vi "VisualizeCHROMAAC.vi"() -> ()   [LabVIEW 2018, in "Visualization.lvlib" / "VisualizeAcPwr.lvclass"]
uses:
  VisualizeAcPwr.lvclass
  VisualizeBase/VisualizeBase_class/Requests/clUserEventType.ctl
  <vilib>/event_ctls.llb/usereventprio.ctl
  <vilib>/Utility/error.llb/Error Cluster From Error Code.vi
  <vilib>/ErrorRing/Error Ring.xnode
  VisualizeBase/VisualizeBase_class/VisualizeBase.lvclass
  <userlib>/NIST/NISTErrorLib/NISTErrorLib.lvlib
  AcPwr/AcPwrModule/AcPwrModule.lvlib
panel:
  in  "GraphAxis":u32[](array[numeric])=[0, 1, 1] max=1
  out "Chroma AC":waveform(dbl)[](graph)
  out "ErrorArray":errorcluster[](array[cluster])
  in  "QueueName":string="CHROMAACVQ"
  in  "btnStop":bool
  in  "btnReset":bool
  in  "btnClear":bool
  # "0=Left Axis and 1=Right Axis"
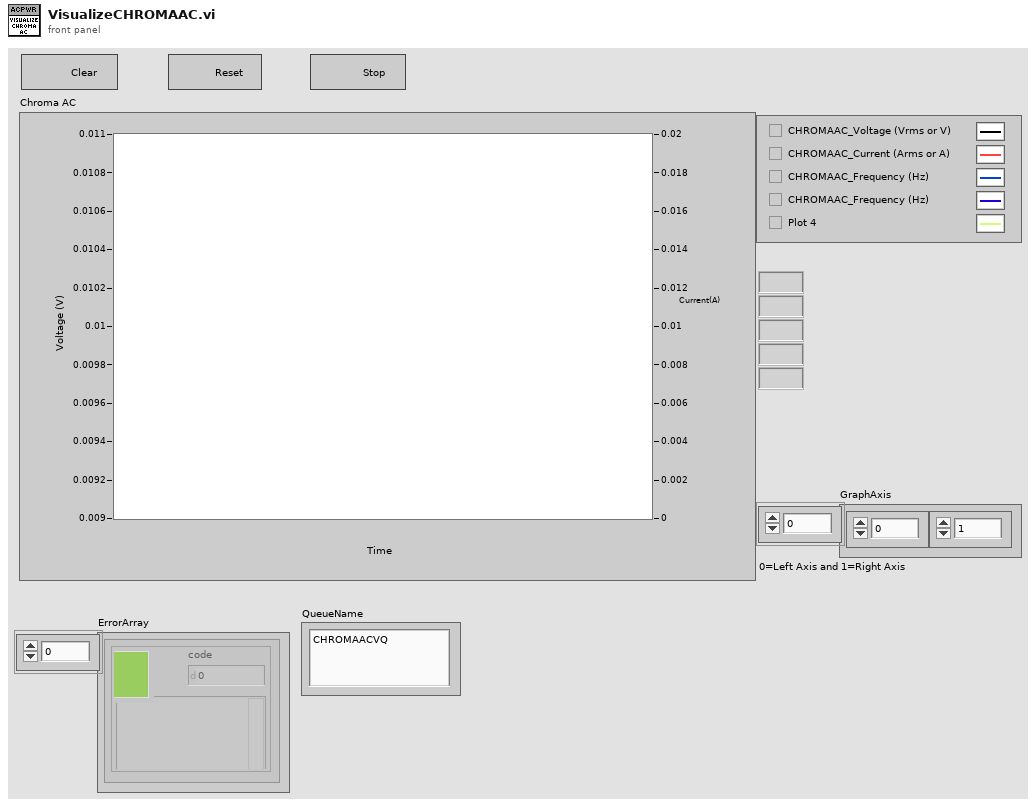
[diagram p1: front panel]
types:
  T1 = typedef "Visualization.lvlib/VisualizeBase.lvclass/clRequestEvents.ctl" = cluster{"StopRequest":refnum<user-event>, "ResetRequest":refnum<user-event>}
  T2 = typedef "AcPwrModule.lvlib/clBroadcastEvents.ctl" = cluster{"DidInit":refnum<user-event>, "StatusUpdate":refnum<user-event>, "ErrorReport":refnum<user-event>, "DidStop":refnum<user-event>, "PathToINI":refnum<user-event>, "Measurements":refnum<user-event>, "LoadConfigFile":refnum<user-event>}
  T3 = typedef "Visualization.lvlib/VisualizeBase.lvclass/clUserEventType.ctl" = cluster{"BusIndex":i8, "Data":variant}
  T4 = typedef "usereventprio.ctl" = enum32{"high priority", "normal priority"}
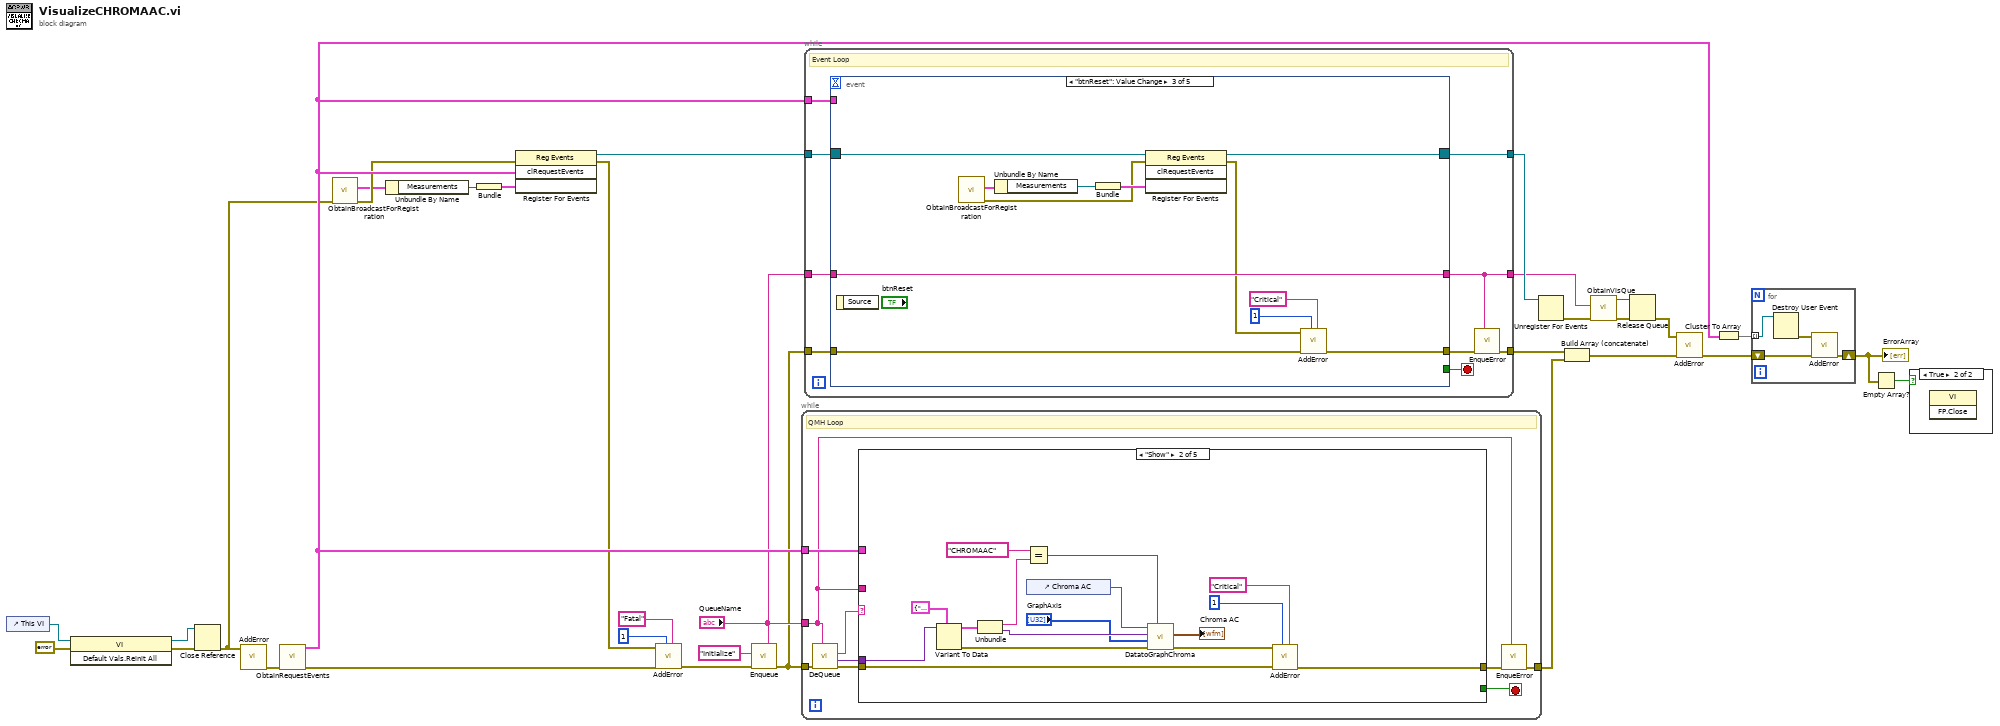
[diagram p0: block diagram]
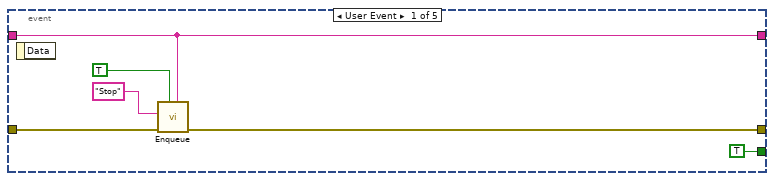
[diagram p2: hidden frame]
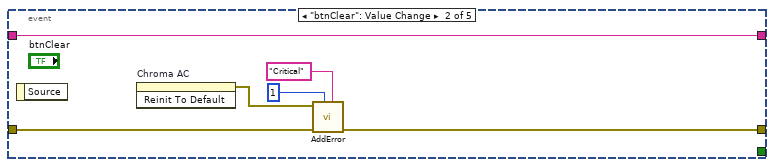
[diagram p3: hidden frame]
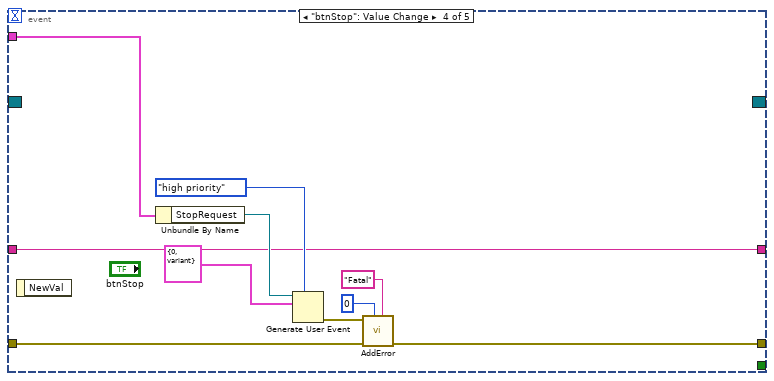
[diagram p4: hidden frame]
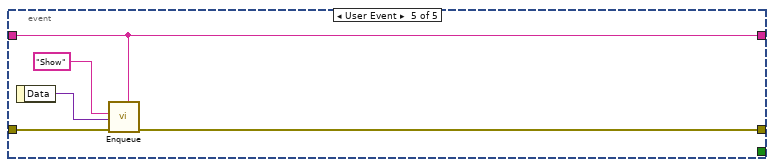
[diagram p5: hidden frame]
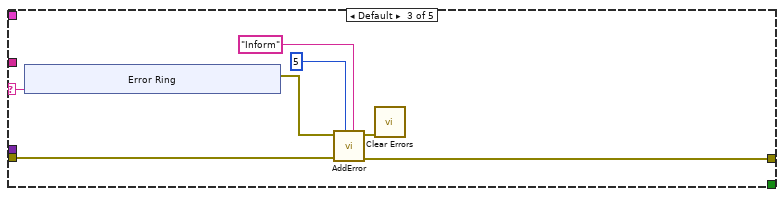
[diagram p8: hidden frame]
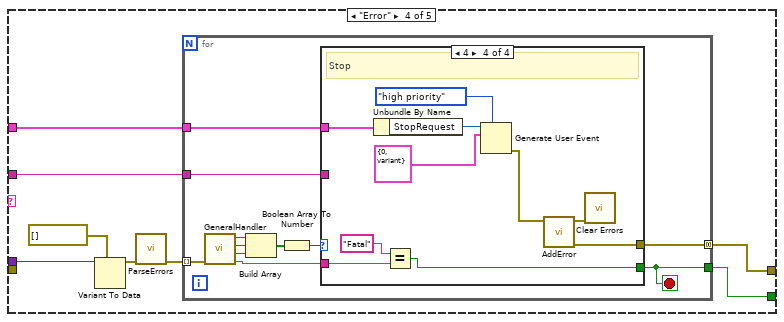
[diagram p9: hidden frame]
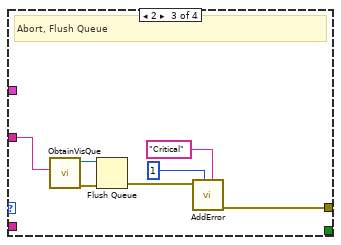
[diagram p12: hidden frame]
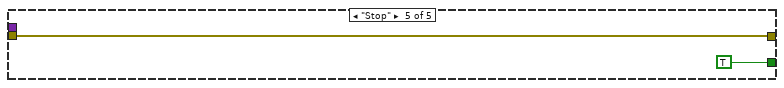
[diagram p13: hidden frame]
diagram:
  n1 = control-ref of="This VI"() -> (w16:refnum<vi>)
  n2 = invoke class="VI" method="Default Vals.Reinit All"(reference=w16, error in=errorcluster {"status"=FALSE, "code"=0, "source"=""} ("error in (no error)")) -> (reference out=w13:refnum<vi>, error out=w14:errorcluster)  [unwired: 1 in, 1 out]
  n3 = Close Reference(reference=w13, error in (no error)=w14) -> (error out=w11:errorcluster)
  n4 = call <userlib>:"AddError.vi"("error in (no error)"=w11) -> ("ErrorArray"=w31:errorcluster[])  [unwired: 9 in, 1 out]
  n5 = call "ObtainRequestEvents.vi"("Error"=w31) -> ("Error"=w4:errorcluster[], "clRequestEvents"=w20:T1)  [unwired: 9 in]
  n6 = call "ObtainBroadcastForRegistration.vi"("error in (no error)"=w11) -> ("error out"=w10:errorcluster, "clBroadcastEvents"=w9:T2)  [unwired: 9 in]
  n7 = Unbundle By Name(w9) -> ("Measurements"=w18:refnum<user-event>)
  n8 = Bundle("Measurements"=w18) -> (w17:cluster{"Measurements":refnum<user-event>})  [unwired: 1 in]
  n9 = register-events(error in=w10, w20, w17) -> (reference out=w32:refnum<event-registration>, error out=w1:errorcluster)  [unwired: 1 in]
  n10 = call <userlib>:"AddError.vi"("Severity"="Fatal" ("String"), "Priority"=u8 1, "ErrorArray"=w4, "error in (no error)"=w1) -> ("ErrorArray"=w3:errorcluster[])  [unwired: 6 in, 1 out]
  n11 = call "Enqueue.vi"("QueName"="QueueName", "Error"=w3, "Message"="Initialize") -> ("Error"=w2:errorcluster[])  [unwired: 8 in]
  n12 = while {
    tunnel: w2 -> [w42]
    tunnel: [w36] -> w27
    tunnel: "QueueName" -> [w34]
    tunnel: w20 -> [w35]
    stop <- w37 stop-if-true
    # "QMH Loop"
    n13 = call "DeQueue.vi"("QueName"=w34, "Error"=w42) -> ("Error"=w39:errorcluster[], "Data"=w40:variant, "Message"=w41:string)  [unwired: 7 in]
    n14 = case shown="\"Show\"" w41 {
      selector: w41 -> [_ _ w66 _ _]
      tunnel: w40 -> [_ w56 _ w81 _]
      tunnel: w39 -> [w43 w48 w64 _ w110]
      tunnel: [w43 w59 w63 w77 w110] -> w38
      tunnel: [_ _ _ w76 TRUE] -> w37
      tunnel: w35 -> [_ _ _ w75 _]
      tunnel: w34 -> [_ _ _ w74 _]
      frame "Initialize" {
      }
      frame "Show" {
        n15 = Variant To Data(type=cluster{string, "Data":variant} {"", "Data"=variant}, Variant=w56) -> (data=w57:cluster{string, "Data":variant}, error out=w51:errorcluster)  [unwired: 1 in]
        n16 = Unbundle(w57) -> (w55:string, "Data"=w52:variant)
        n17 = Equal?(x="CHROMAAC", y=w55) -> (x = y?=w49:bool)
        n18 = control-ref of="Chroma AC"() -> (w54:refnum<vi>)
        n19 = call "DatatoGraphChroma.vi"("Boolean"=w49, "error in (no error)"=w51, "Array 2"="GraphAxis", "Data"=w52, "WaveformChart in"=w54) -> ("error out"=w46:errorcluster, "Array"=→"Chroma AC":waveform(dbl)[])  [unwired: 3 in, 2 out]
        n20 = call <userlib>:"AddError.vi"("Severity"="Critical" ("String"), "Priority"=u8 1, "ErrorArray"=w48, "error in (no error)"=w46) -> ("ErrorArray"=w59:errorcluster[])  [unwired: 6 in, 1 out]
      }
      frame Default {
        n21 = xnode "Error Ring"("parameter 0"=w66) -> ("error out"=w65:errorcluster)
        n22 = call <userlib>:"AddError.vi"("Severity"="Inform" ("String"), "Priority"=u8 5, "ErrorArray"=w64, "error in (no error)"=w65) -> ("ErrorArray"=w63:errorcluster[], "error out"=w62:errorcluster)  [unwired: 6 in]
        n23 = call <vilib>:"Clear Errors.vi"("error in (no error)"=w62) -> ()  [unwired: 5 in, 2 out]
      }
      frame "Error" {
        n24 = Variant To Data(type=errorcluster[] [], Variant=w81) -> (data=w79:errorcluster[])  [unwired: 1 in, 1 out]
        n25 = call <userlib>:"ParseErrors.vi"("ErrorArray"=w79) -> ("ErrorArray"=w78:errorcluster[])  [unwired: 8 in, 2 out]
        n26 = for {
          tunnel: w78 -> [w92] mode=indexing
          tunnel: [w86] -> w77 mode=concatenating
          tunnel: [w84] -> w76
          tunnel: w75 -> [w83]
          tunnel: w74 -> [w82]
          stop <- w84 stop-if-true
          n27 = call <userlib>:"GeneralHandler.vi"("error in (no error)"=w92) -> ("Severity"=w85:string, "Stop"=w89:bool, "Abort"=w90:bool, "Continue"=w91:bool)  [unwired: 7 in]
          n28 = Build Array(w91, w90, w89) -> (w88:bool[])
          n29 = Boolean Array To Number(Boolean array=w88) -> (number=w87:u32)
          n30 = case shown="4" w87 {
            tunnel: [_ _ w97 w108] -> w86
            tunnel: w85 -> [_ _ _ w103]
            tunnel: [_ _ _ w101] -> w84
            tunnel: w83 -> [_ _ _ w100]
            tunnel: w82 -> [_ _ w93 _]
            frame 0, Default {
              # "No Dialog"
            }
            frame 1 {
              # "Continue"
            }
            frame 2 {
              # "Abort, Flush Queue"
              n31 = call "ObtainVisQue.vi"("QueName"=w93) -> ("error out"=w99:errorcluster, "queue out"=w98:refnum<queue>)  [unwired: 9 in]
              n32 = Flush Queue(queue=w98, error in (no error)=w99) -> (error out=w96:errorcluster)  [unwired: 2 out]
              n33 = call <userlib>:"AddError.vi"("Severity"="Critical" ("String"), "Priority"=u8 1, "error in (no error)"=w96) -> ("ErrorArray"=w97:errorcluster[])  [unwired: 7 in, 1 out]
            }
            frame 4 {
              # "Stop"
              n34 = Unbundle By Name(w100) -> ("StopRequest"=w109:refnum<user-event>)
              n35 = Equal?(x="Fatal", y=w103) -> (x = y?=w101:bool)
              n36 = Generate User Event(priority (normal)=usereventprio."high priority", user event=w109, event data cluster=T3 {"BusIndex"=0, "Data"=variant} ("event data")) -> (error out=w107:errorcluster)  [unwired: 1 in, 1 out]
              n37 = call <userlib>:"AddError.vi"("error in (no error)"=w107) -> ("ErrorArray"=w108:errorcluster[], "error out"=w104:errorcluster)  [unwired: 9 in]
              n38 = call <vilib>:"Clear Errors.vi"("error in (no error)"=w104) -> ()  [unwired: 5 in, 2 out]
            }
          }
        }
      }
      frame "Stop" {
      }
    }
    n39 = call "EnqueError.vi"("QueName"=w34, "Error"=w38) -> ("Error"=w36:errorcluster[])  [unwired: 9 in]
  }
  n40 = while {
    tunnel: w32 -> [w120]
    tunnel: [w117] -> w28
    tunnel: [w116] -> w30
    tunnel: w20 -> [w115]
    tunnel: w2 -> [w114]
    tunnel: "QueueName" -> [w113]
    tunnel: [w112] -> w7
    stop <- w119 stop-if-true
    # "Event Loop"
    n41 = event shown="[2] \"btnReset\": Value Change" {
      selector: w120 -> [_ _ w144 _ _]
      dyn-events: [_ _ w143 _ _] -> w116
      timeout: _ -> [_ _ _ _ _]
      tunnel: [TRUE _ _ _ _] -> w119
      tunnel: [w125 w128 w136 w152 w157] -> w118
      tunnel: w115 -> [_ _ _ w147 _]
      tunnel: w114 -> [w121 w129 w137 w145 w155]
      tunnel: w113 -> [w122 w132 w138 w146 w156]
      tunnel: [w122 w132 w138 w146 w156] -> w112
      event User Event {
        n42 = event-data() -> ()  [unwired: 1 in, 1 out]
        n43 = call "Enqueue.vi"("QueName"=w122, "Priority? (F)"=TRUE, "Error"=w121, "Message"="Stop") -> ("Error"=w125:errorcluster[])  [unwired: 7 in]
      }
      event "btnClear": Value Change {
        n44 = event-data() -> ()  [unwired: 1 in, 1 out]
        n45 = invoke on="Chroma AC" class="WFChart (strict)" method="Reinit To Default"() -> (error out=w127:errorcluster)  [unwired: 3 in, 2 out]
        n46 = call <userlib>:"AddError.vi"("Severity"="Critical" ("String"), "Priority"=u8 1, "ErrorArray"=w129, "error in (no error)"=w127) -> ("ErrorArray"=w128:errorcluster[])  [unwired: 6 in, 1 out]
      }
      event "btnReset": Value Change {
        n47 = event-data() -> ()  [unwired: 1 in, 1 out]
        n48 = call "ObtainBroadcastForRegistration.vi"() -> ("error out"=w139:errorcluster, "clBroadcastEvents"=w140:T2)  [unwired: 10 in]
        n49 = Unbundle By Name(w140) -> ("Measurements"=w142:refnum<user-event>)
        n50 = Bundle("Measurements"=w142) -> (w141:cluster{"Measurements":refnum<user-event>})  [unwired: 1 in]
        n51 = register-events(reference=w144, error in=w139, w141) -> (reference out=w143:refnum<event-registration>, error out=w135:errorcluster)  [unwired: 1 in]
        n52 = call <userlib>:"AddError.vi"("Severity"="Critical" ("String"), "Priority"=u8 1, "ErrorArray"=w137, "error in (no error)"=w135) -> ("ErrorArray"=w136:errorcluster[])  [unwired: 6 in, 1 out]
      }
      event "btnStop": Value Change {
        n53 = event-data() -> ()  [unwired: 1 in, 1 out]
        n54 = Unbundle By Name(w147) -> ("StopRequest"=w153:refnum<user-event>)
        n55 = Generate User Event(priority (normal)=usereventprio."high priority", user event=w153, event data cluster=T3 {"BusIndex"=0, "Data"=variant} ("event data")) -> (error out=w154:errorcluster)  [unwired: 1 in, 1 out]
        n56 = call <userlib>:"AddError.vi"("Severity"="Fatal" ("String"), "Priority"=u8 0, "ErrorArray"=w145, "error in (no error)"=w154) -> ("ErrorArray"=w152:errorcluster[])  [unwired: 6 in, 1 out]
      }
      event User Event {
        n57 = event-data() -> ("Data"=w159:variant)  [unwired: 1 in]
        n58 = call "Enqueue.vi"("QueName"=w156, "Error"=w155, "Data"=w159, "Message"="Show") -> ("Error"=w157:errorcluster[])  [unwired: 7 in]
      }
    }
    n59 = call "EnqueError.vi"("QueName"=w112, "Error"=w118) -> ("Error"=w117:errorcluster[])  [unwired: 9 in]
  }
  n60 = Unregister For Events(event registration refnum=w30) -> (error out=w26:errorcluster)  [unwired: 1 in]
  n61 = Build Array (concatenate)(w28, w27) -> (w25:errorcluster[])
  n62 = call "ObtainVisQue.vi"("error in (no error)"=w26, "QueName"=w7) -> ("error out"=w24:errorcluster, "queue out"=w23:refnum<queue>)  [unwired: 8 in]
  n63 = Release Queue(queue=w23, error in (no error)=w24) -> (error out=w22:errorcluster)  [unwired: 1 in, 2 out]
  n64 = call <userlib>:"AddError.vi"("ErrorArray"=w25, "error in (no error)"=w22) -> ("ErrorArray"=w21:errorcluster[])  [unwired: 8 in, 1 out]
  n65 = Cluster To Array(cluster=w20) -> (array=w29:refnum<user-event>[])
  n66 = for {
    tunnel: w29 -> [w163] mode=indexing
    shift-right: [w162] -> w12
    shift-left: w21 -> [w161]
    n67 = Destroy User Event(user event=w163) -> (error out=w160:errorcluster)  [unwired: 1 in]
    n68 = call <userlib>:"AddError.vi"("ErrorArray"=w161, "error in (no error)"=w160) -> ("ErrorArray"=w162:errorcluster[])  [unwired: 8 in, 1 out]
  }
  "ErrorArray" <- w12
  n69 = Empty Array?(array=w12) -> (empty?=w19:bool)
  n70 = case shown="True" w19 {
    frame False {
    }
    frame True {
      n71 = invoke class="VI" method="FP.Close"() -> ()  [unwired: 3 in, 3 out]
    }
  }
